vi "PNEU_Ref_Num.vi"() -> (0 "Pneu":T1)   [LabVIEW 2015]
uses:
  Pneu_Type_Def.ctl
  <vilib>/Rock Robotics/WPI/Solenoid/WPI_SolenoidDevRef.ctl
  <vilib>/Rock Robotics/WPI/Solenoid/WPI_SolenoidChannel.ctl
  <vilib>/Rock Robotics/WPI/Compressor/WPI_CompressorDevRef.ctl
  <vilib>/Rock Robotics/WPI/Utilities/WPI_GetSetVariantRefNum.vi
panel:
  # "Nick Nannen"
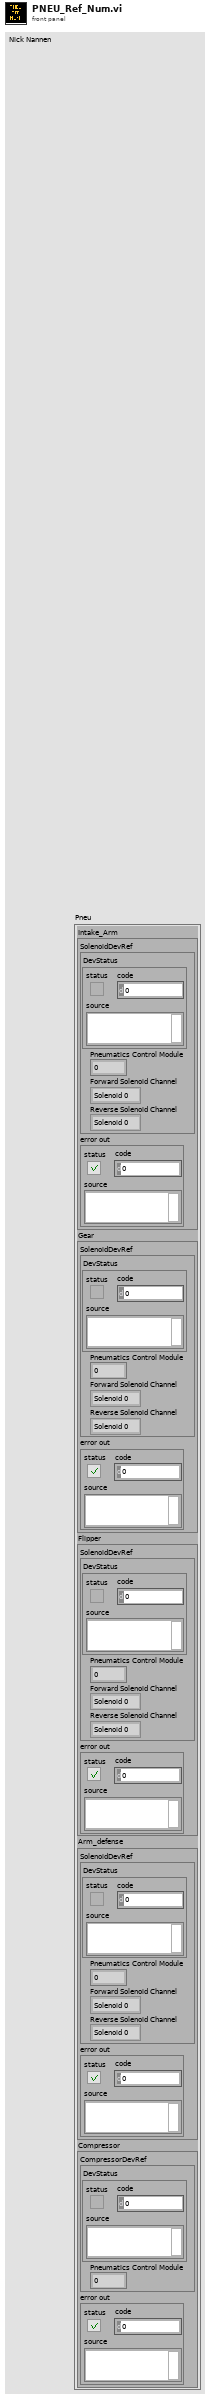
[diagram p1: front panel]
types:
  T1 = typedef "Pneu_Type_Def.ctl" = cluster{"Intake_Arm":cluster{"SolenoidDevRef":T2, "error out":errorcluster}, "Gear":cluster{"SolenoidDevRef":T2, "error out":errorcluster}, "Flipper":cluster{"SolenoidDevRef":T2, "error out":errorcluster}, "Arm_defense":cluster{"SolenoidDevRef":T2, "error out":errorcluster}, "Compressor":cluster{"CompressorDevRef":T4, "error out":errorcluster}}
  T2 = typedef "WPI_SolenoidDevRef.ctl" = cluster{"DevStatus":errorcluster, "Pneumatics Control Module":u8, "Forward Solenoid Channel":T3, "Reverse Solenoid Channel":T3}
  T3 = typedef "WPI_SolenoidChannel.ctl" = enum8{"Solenoid 0", "Solenoid 1", "Solenoid 2", "Solenoid 3", "Solenoid 4", "Solenoid 5", "Solenoid 6", "Solenoid 7", "Invalid"}
  T4 = typedef "WPI_CompressorDevRef.ctl" = cluster{"DevStatus":errorcluster, "Pneumatics Control Module":u8}
  T5 = cluster{"CompressorDevRef":T4, "error out":errorcluster}
  T6 = cluster{"SolenoidDevRef":T2, "error out":errorcluster}
  T7 = cluster{"Intake_Arm":cluster{"SolenoidDevRef":T2, "error out":errorcluster}, "Gear":cluster{"SolenoidDevRef":T2, "error out":errorcluster}, "Flipper":cluster{"SolenoidDevRef":T2, "error out":errorcluster}, "Arm_defense":cluster{"SolenoidDevRef":T2, "error out":errorcluster}, "Compressor":cluster{"CompressorDevRef":T4, "error out":errorcluster}}
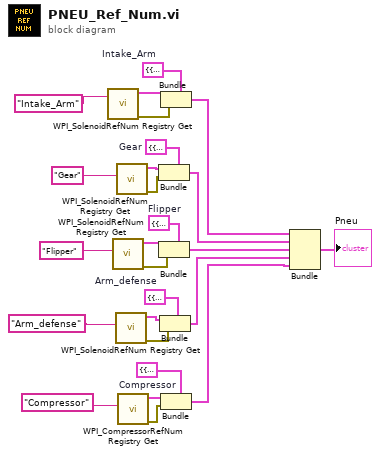
[diagram p0: block diagram]
diagram:
  w2 = T5 {"CompressorDevRef"={"DevStatus"={"status"=FALSE, "code"=0, "source"=""}, "Pneumatics Control Module"=0}, "error out"={"status"=FALSE, "code"=0, "source"=""}}  # Compressor
  w6 = T6 {"SolenoidDevRef"={"DevStatus"={"status"=FALSE, "code"=0, "source"=""}, "Pneumatics Control Module"=0, "Forward Solenoid Channel"=enum."Solenoid 0", "Reverse Solenoid Channel"=enum."Solenoid 0"}, "error out"={"status"=FALSE, "code"=0, "source"=""}}  # Arm_defense
  w8 = T6 {"SolenoidDevRef"={"DevStatus"={"status"=FALSE, "code"=0, "source"=""}, "Pneumatics Control Module"=0, "Forward Solenoid Channel"=enum."Solenoid 0", "Reverse Solenoid Channel"=enum."Solenoid 0"}, "error out"={"status"=FALSE, "code"=0, "source"=""}}  # Flipper
  w9 = T6 {"SolenoidDevRef"={"DevStatus"={"status"=FALSE, "code"=0, "source"=""}, "Pneumatics Control Module"=0, "Forward Solenoid Channel"=enum."Solenoid 0", "Reverse Solenoid Channel"=enum."Solenoid 0"}, "error out"={"status"=FALSE, "code"=0, "source"=""}}  # Gear
  w10 = T6 {"SolenoidDevRef"={"DevStatus"={"status"=FALSE, "code"=0, "source"=""}, "Pneumatics Control Module"=0, "Forward Solenoid Channel"=enum."Solenoid 0", "Reverse Solenoid Channel"=enum."Solenoid 0"}, "error out"={"status"=FALSE, "code"=0, "source"=""}}  # Intake_Arm
  n1 = call <vilib>:"WPI_SolenoidRefNum Registry Get.vi"("refnum name"="Intake_Arm") -> ("error out"=w20:errorcluster, "SolenoidDevRef"=w21:T2)  [unwired: 9 in]
  n2 = call <vilib>:"WPI_SolenoidRefNum Registry Get.vi"("refnum name"="Flipper") -> ("error out"=w14:errorcluster, "SolenoidDevRef"=w15:T2)  [unwired: 9 in]
  n3 = call <vilib>:"WPI_SolenoidRefNum Registry Get.vi"("refnum name"="Arm_defense") -> ("error out"=w12:errorcluster, "SolenoidDevRef"=w13:T2)  [unwired: 9 in]
  n4 = call <vilib>:"WPI_SolenoidRefNum Registry Get.vi"("refnum name"="Gear") -> ("error out"=w17:errorcluster, "SolenoidDevRef"=w18:T2)  [unwired: 9 in]
  n5 = call <vilib>:"WPI_CompressorRefNum Registry Get.vi"("refnum name"="Compressor") -> ("error out"=w3:errorcluster, "CompressorDevRef"=w4:T4)  [unwired: 9 in]
  n6 = Bundle(cluster=w9, "SolenoidDevRef"=w18, "error out"=w17) -> (w25:T6)
  n7 = Bundle(cluster=w8, "SolenoidDevRef"=w15, "error out"=w14) -> (w24:T6)
  n8 = Bundle(cluster=w6, "SolenoidDevRef"=w13, "error out"=w12) -> (w23:T6)
  n9 = Bundle(cluster=w10, "SolenoidDevRef"=w21, "error out"=w20) -> (w26:T6)
  n10 = Bundle(cluster=w2, "CompressorDevRef"=w4, "error out"=w3) -> (w22:T5)
  n11 = Bundle("Intake_Arm"=w26, "Gear"=w25, "Flipper"=w24, "Arm_defense"=w23, "Compressor"=w22) -> (→"Pneu":T7)  [unwired: 1 in]
